vi "Save Data.vi"(8 "error in (no error)":errorcluster, 11 "Micron sm Digitizer in":refnum<class "Micron sm Digitizer.lvclass">) -> (0 "error out":errorcluster, 1 "Finished":bool, 2 "Current read position":i32, 3 "Micron sm Digitizer out":refnum<class "Micron sm Digitizer.lvclass">)   [LabVIEW 2024, in "Micron sm Digitizer.lvclass"]
uses:
  Micron sm Digitizer.lvclass
  Micron sm Digitizer.lvclass/Micron sm Digitizer.ctl
  Micron Optics sm130/Micron Optics sm130.lvlib
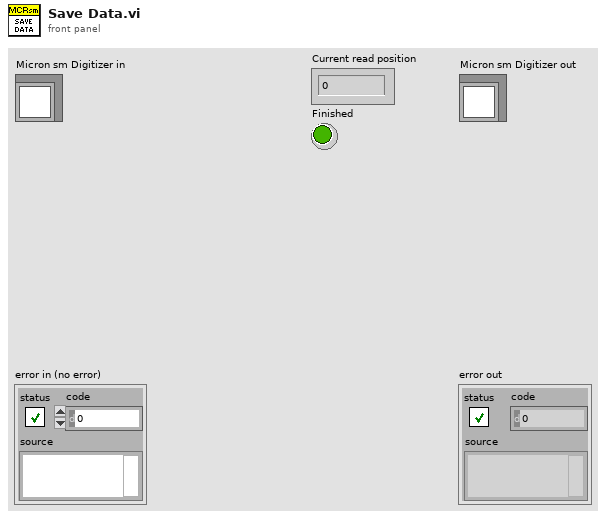
[diagram p1: front panel]
types:
  T1 = cluster{"Data Serial Number":u32, "Time Stamp":dbl, "Sub-Channel":u8}
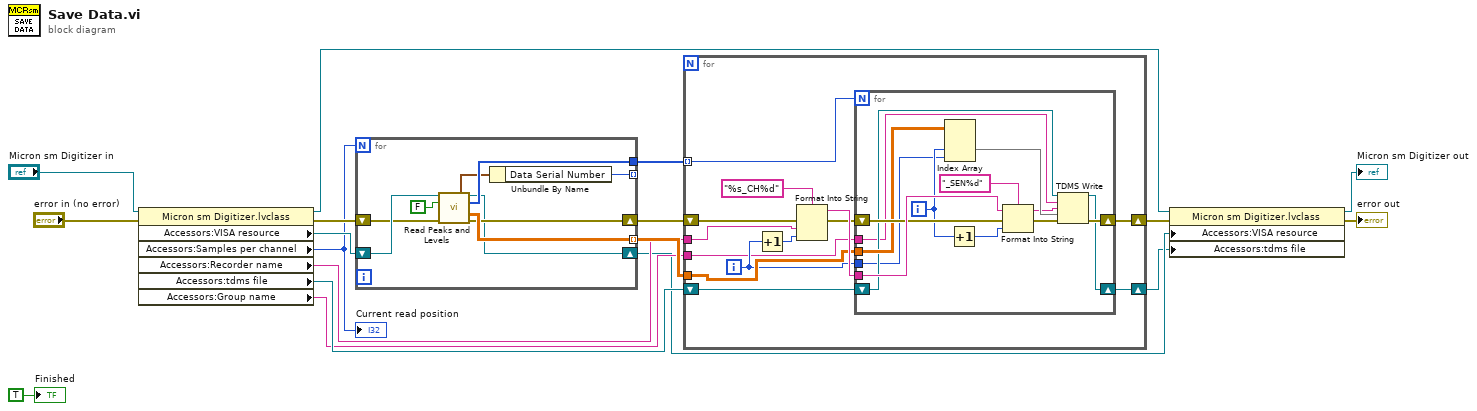
[diagram p0: block diagram]
diagram:
  n1 = property class="Micron sm Digitizer.lvclass"(reference="Micron sm Digitizer in", error in="error in (no error)") -> (reference out=w5:refnum<class "Micron sm Digitizer.lvclass">, error out=w15:errorcluster, "Accessors:VISA resource"=w16:refnum<visa-resource-name>, "Accessors:Samples per channel"=w1:i32, "Accessors:Recorder name"=w12:string, "Accessors:tdms file"=w10:refnum<k34>, "Accessors:Group name"=w9:string)
  "Current read position" <- w1
  n2 = for {
    N: w1 -> [_]
    tunnel: [w25] -> w14
    tunnel: [w24] -> w13 mode=indexing
    shift-right: [w23] -> w11
    shift-left: w15 -> [w26]
    shift-right: [w22] -> w8
    shift-left: w16 -> [w27]
    tunnel: [w20] -> _ mode=indexing
    n3 = call "Read Peaks and Levels.vi"("VISA resource name"=w27, "Enable Unbuffered Data (Enabled)"=FALSE, "error in (no error)"=w26) -> ("Data Status"=w21:T1, "VISA resource name out"=w22:refnum<visa-resource-name>, "Number of Sensors"=w25:u16[], "Peak Wavelengths (nm)"=w24:dbl[][], "error out"=w23:errorcluster)  [unwired: 4 in, 4 out]
    n4 = Unbundle By Name(w21) -> ("Data Serial Number"=w20:u32)
  }
  n5 = for {
    tunnel: w14 -> [w40] mode=indexing
    tunnel: w13 -> [w32]
    tunnel: w12 -> [w38]
    shift-right: [w33] -> w4
    shift-left: w11 -> [w35]
    tunnel: w9 -> [w29]
    shift-right: [w28] -> w7
    shift-left: w10 -> [w30]
    i -> [w31]
    n6 = Increment(x=w31) -> (x+1=w37:i32)
    n7 = Format Into String(format string="%s_CH%d", error in=w35, w38, w37) -> (resulting string=w36:string, error out=w34:errorcluster)  [unwired: 1 in]
    n8 = for {
      N: w40 -> [_]
      tunnel: w36 -> [w54]
      shift-right: [w43] -> w33
      shift-left: w34 -> [w52]
      tunnel: w32 -> [w50]
      tunnel: w31 -> [w41]
      tunnel: w29 -> [w46]
      shift-right: [w42] -> w28
      shift-left: w30 -> [w48]
      i -> [w49]
      n9 = Index Array(array=w50, index (dim 1)=w49, index (dim 2)=w41) -> (element=w45:dbl[])  [unwired: 1 in]
      n10 = Increment(x=w49) -> (x+1=w51:i32)
      n11 = Format Into String(format string="_SEN%d", initial string=w54, error in=w52, w51) -> (resulting string=w44:string, error out=w47:errorcluster)
      n12 = TDMS Write(0:w48, 5:w46, 7:w44, 9:w45, 11:w47) -> (4:w42:refnum<k34>, 15:w43:errorcluster)  [unwired: 1 in, 2 out]
    }
  }
  n13 = property class="Micron sm Digitizer.lvclass"(reference=w5, error in=w4, "Accessors:VISA resource"=w8, "Accessors:tdms file"=w7) -> (reference out=→"Micron sm Digitizer out":refnum<class "Micron sm Digitizer.lvclass">, error out=→"error out":errorcluster)
  "Finished" <- TRUE ("Finished")
